vi "Read Button Properties.vi"(8 "error in (no error)":errorcluster, 11 "ButtonControlEditorPanel in":refnum<class "ButtonControlEditorPanel.lvclass">) -> (0 "error out":errorcluster, 2 "output cluster":T1, 3 "ButtonControlEditorPanel out":refnum<class "ButtonControlEditorPanel.lvclass">)   [LabVIEW 2020, in "VolatusGUIControls.lvlib" / "ButtonControlEditorPanel.lvclass"]
uses:
  ButtonControlEditorPanel.lvclass
  ButtonControlEditorPanel.lvclass/ButtonControlEditorPanel.ctl
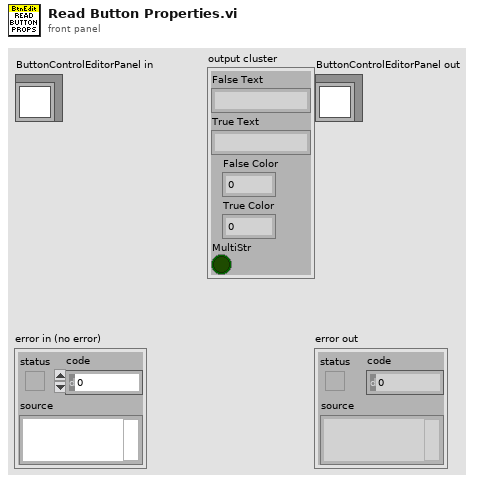
[diagram p1: front panel]
types:
  T1 = cluster{"False Text":string, "True Text":string, "False Color":u32, "True Color":u32, "MultiStr":bool}
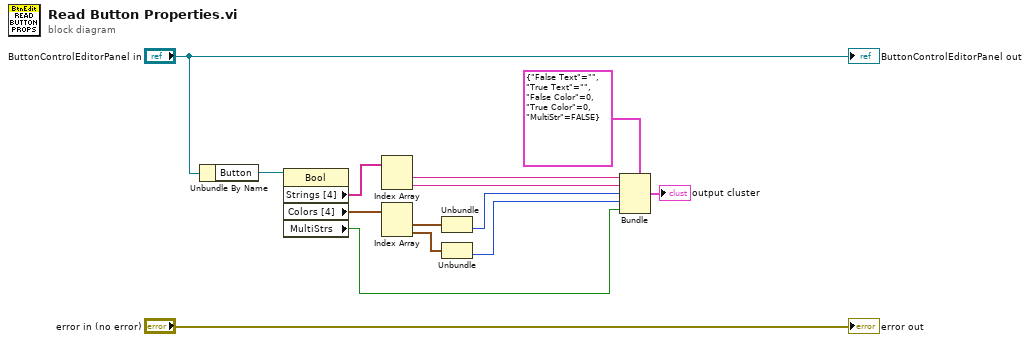
[diagram p0: block diagram]
diagram:
  n1 = Unbundle By Name("ButtonControlEditorPanel in") -> ("Button"=w12:refnum<vi>)
  n2 = property class="Bool"(reference=w12) -> ("Strings [4]"=w11:string[], "Colors [4]"=w10:cluster{u32, u32}[], "MultiStrs"=w1:bool)  [unwired: 1 in, 2 out]
  n3 = Index Array(array=w11) -> (element #1=w6:string, element #2=w5:string)  [unwired: 2 in]
  n4 = Index Array(array=w10) -> (element #1=w9:cluster{u32, u32}, element #2=w8:cluster{u32, u32})  [unwired: 2 in]
  n5 = Unbundle(w9) -> (w4:u32)  [unwired: 1 out]
  n6 = Unbundle(w8) -> (w3:u32)  [unwired: 1 out]
  n7 = Bundle(cluster=T1 {"False Text"="", "True Text"="", "False Color"=0, "True Color"=0, "MultiStr"=FALSE}, "False Text"=w6, "True Text"=w5, "False Color"=w4, "True Color"=w3, "MultiStr"=w1) -> (→"output cluster":T1)
  "error out" <- "error in (no error)"
  "ButtonControlEditorPanel out" <- "ButtonControlEditorPanel in"
